vi "SubDaqWork.vi"(8 "error in (no error)":errorcluster, 9 "SubQueueIN":refnum<queue>, 10 "MainQueueIN":refnum<queue>, 11 "Data Value Reference IN":refnum<data-value>) -> (0 "error out":errorcluster, 3 "Data Value Reference out":refnum<data-value>)   [LabVIEW 2013]
uses:
  Control/SystemCommand.ctl
  Control/SystemData.ctl
  Control/SignalType.ctl
  Control/SubDaqCommand.ctl
  <vilib>/measure/NI_MABase.lvlib
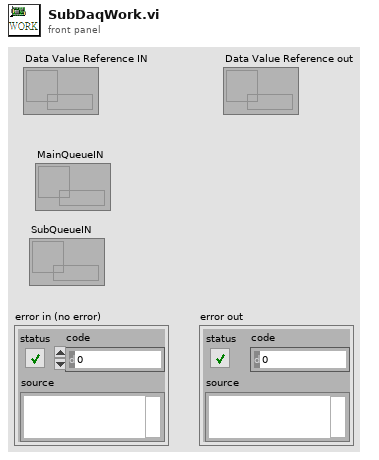
[diagram p1: front panel]
types:
  T1 = typedef "SubDaqCommand.ctl" = enum16{"None", "Init", "Work", "Stop", "Close"}
  T2 = enum16{"Sine Wave", "Triangle Wave", "Square Wave", "Sawtooth Wave"}
  T3 = typedef "SystemCommand.ctl" = enum16{"None", "Init", "Close", "ShowNumeric", "ShowString", "ShowBool", "SquareNumeric", "ReverseString", "InvertBool", "FFT"}
  T4 = typedef "SystemData.ctl" = cluster{"Numeric":dbl, "String":string, "Boolean":bool, "Frequency":dbl, "Amplitude":dbl, "SignalType":T5, "WaveformArray":waveform(dbl)[], "Reset":bool, "StateString":string, "FFTmagnitudes":cluster{"f0":dbl, "df":dbl, "magnitude":dbl[]}[]}
  T5 = typedef "SignalType.ctl" = enum16{"Sin", "Triangle", "Square"}
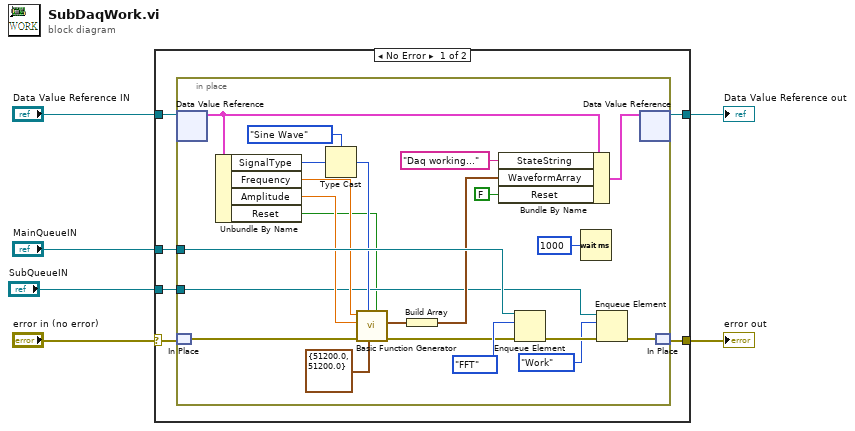
[diagram p0: block diagram]
diagram:
  n1 = case shown="No Error" "error in (no error)" {
    selector: "error in (no error)" -> [w10 w35]
    tunnel: "Data Value Reference IN" -> [w12 w36]
    tunnel: [w11 w36] -> w3
    tunnel: [w9 w35] -> w5
    tunnel: "MainQueueIN" -> [w8 _]
    tunnel: "SubQueueIN" -> [w7 _]
    frame No Error {
      n2 = in-place {
        in-place-border: w8 -> [w34]
        in-place-border: w7 -> [w20]
        n3 = in-place-dvr #1(w12) -> (w22:T4)  [unwired: 1 out]
        n4 = in-place-match #2(w10) -> (w32:errorcluster)
        n5 = Unbundle By Name(w22) -> ("SignalType"=w26:T5, "Frequency"=w29:dbl, "Amplitude"=w28:dbl, "Reset"=w15:bool)
        n6 = Type Cast(type=T2."Sine Wave" ("signal type"), x=w26) -> (*(type *) &x=w25:T2)
        n7 = call <vilib>:"Basic Function Generator.vi"("reset signal"=w15, "sampling info"=cluster{"Fs":dbl, "#s":dbl} {"Fs"=51200.0, "#s"=51200.0}, "signal type"=w25, "error in (no error)"=w32, "amplitude"=w28, "frequency"=w29) -> ("error out"=w31:errorcluster, "signal out"=w24:waveform(dbl))  [unwired: 3 in, 1 out]
        n8 = Build Array(w24) -> (w23:waveform(dbl)[])
        n9 = Bundle By Name(cluster=w22, "StateString"="Daq working...", "WaveformArray"=w23, "Reset"=FALSE) -> (w21:T4)
        n10 = Enqueue Element(queue=w34, element=SystemCommand."FFT" ("Command"), error in (no error)=w31) -> (error out=w19:errorcluster)  [unwired: 1 in, 2 out]
        n11 = Wait (ms)(milliseconds to wait=u32 1000) -> ()  [unwired: 1 out]
        n12 = Enqueue Element(queue=w20, element=SubDaqCommand."Work", error in (no error)=w19) -> (error out=w18:errorcluster)  [unwired: 1 in, 2 out]
        n13 = in-place-dvr #1(w21) -> (w11:refnum<data-value>)  [unwired: 1 out]
        n14 = in-place-match #2(w18) -> (w9:errorcluster)
      }
    }
    frame Error {
    }
  }
  "error out" <- w5
  "Data Value Reference out" <- w3
